vi "testing.vi"() -> ()   [LabVIEW 2014]
panel:
  out "variant":variant
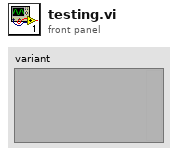
[diagram p1: front panel]
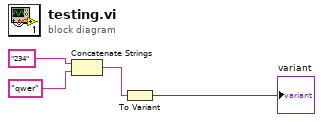
[diagram p0: block diagram]
diagram:
  n1 = Concatenate Strings("234", "qwer") -> (w1:string)
  n2 = To Variant(anything=w1) -> (Variant=→"variant":variant)
